vi "1-BlinkingLED.vi"() -> ()   [LabVIEW 2019]
panel:
  in  "?":bool
  in  "LED OFF time in ms":u32=1000
  in  "LED ON time in ms":u32=1000
  out "?":bool=TRUE
  # "Blinking LED"
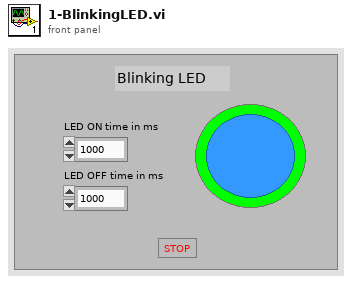
[diagram p1: front panel]
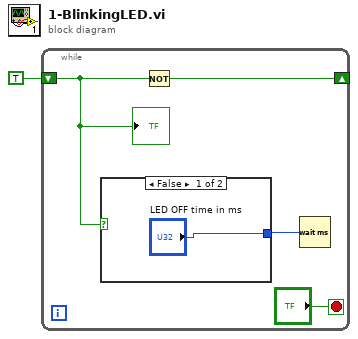
[diagram p0: block diagram]
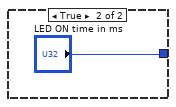
[diagram p2: hidden frame]
diagram:
  n1 = while {
    shift-right: [w5] -> _
    shift-left: TRUE -> [w3]
    stop <- "?" stop-if-true
    n2 = case shown="False" w3 {
      tunnel: ["LED OFF time in ms" "LED ON time in ms"] -> w4
      frame False {
      }
      frame True {
      }
    }
    n3 = Not(x=w3) -> (.not. x?=w5:bool)
    n4 = Wait (ms)(milliseconds to wait=w4) -> ()  [unwired: 1 out]
    "?" <- w3
  }
